vi "Restore Framework.vi"(10 "Files and Folders":path[](array[path])) -> (0 "error out":errorcluster)   [LabVIEW 2025]
uses:
  <vilib>/zip/NI_Unzip.lvlib
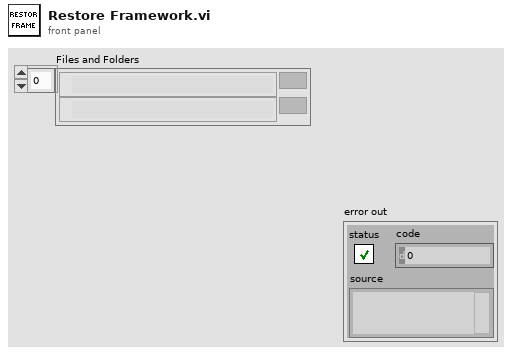
[diagram p1: front panel]
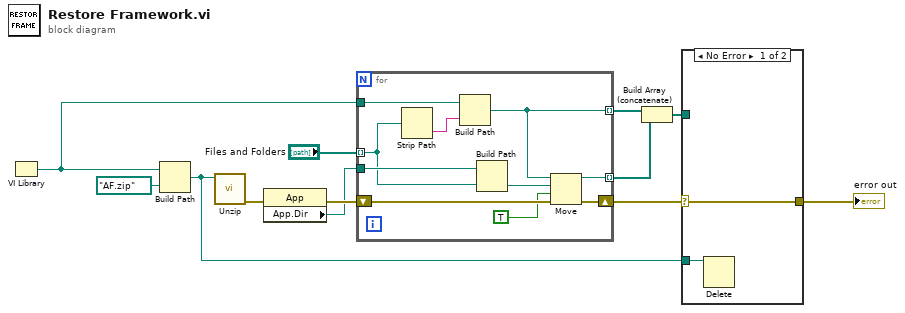
[diagram p0: block diagram]
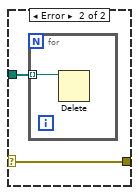
[diagram p2: hidden frame]
diagram:
  n1 = VI Library() -> (path=w9:path)
  n2 = Build Path(base path=w9, name or relative path=path "AF.zip") -> (appended path=w2:path)
  n3 = call <vilib>:"Unzip.vi"("Zip file"=w2) -> ("error out"=w11:errorcluster)  [unwired: 8 in, 2 out]
  n4 = property class="App"(error in=w11) -> (error out=w10:errorcluster, "App.Dir"=w7:path)  [unwired: 1 in, 1 out]
  n5 = for {
    tunnel: w9 -> [w21]
    shift-right: [w20] -> w3
    shift-left: w10 -> [w22]
    tunnel: "Files and Folders" -> [w17] mode=indexing
    tunnel: w7 -> [w18]
    tunnel: [w14] -> w6 mode=indexing
    tunnel: [w13] -> w4 mode=indexing
    n6 = Strip Path(path=w17) -> (name=w16:string)  [unwired: 1 out]
    n7 = Build Path(base path=w21, name or relative path=w16) -> (appended path=w14:path)
    n8 = Build Path(base path=w18, name or relative path=w17) -> (appended path=w19:path)
    n9 = Move(source path=w14, error in=w22, 9:TRUE ("overwrite (F)"), 10:w19) -> (error out=w20:errorcluster, 3:w13:path)  [unwired: 1 in, 1 out]
  }
  n10 = Build Array (concatenate)(w6, w4) -> (w5:path[])
  n11 = case shown="No Error" w3 {
    selector: w3 -> [w23 w25]
    tunnel: w5 -> [_ w26]
    tunnel: [w23 w25] -> w1
    tunnel: w2 -> [w24 _]
    frame No Error {
      n12 = Delete(path (use dialog)=w24) -> ()  [unwired: 4 in, 3 out]
    }
    frame Error {
      n13 = for {
        tunnel: w26 -> [w27] mode=indexing
        n14 = Delete(path (use dialog)=w27) -> ()  [unwired: 4 in, 3 out]
      }
    }
  }
  "error out" <- w1
